vi "BoilerTimer.vi"(8 "error in (no error)":errorcluster, 10 "Enum":T1, 11 "Timer in":dbl) -> (0 "error out":errorcluster, 2 "Timer Up":bool, 3 "Elapsed Time":dbl)   [LabVIEW 2020]
uses:
  BoilerTimerStates.ctl
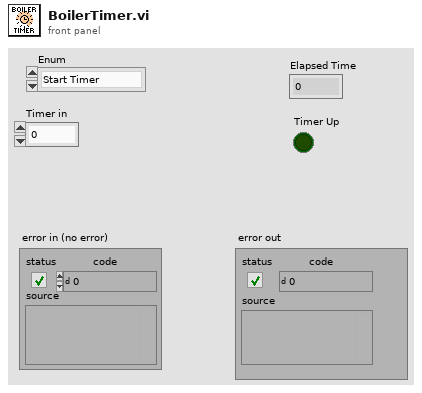
[diagram p1: front panel]
types:
  T1 = typedef "BoilerTimerStates.ctl" = enum16{"Start Timer", "Check Timer"}
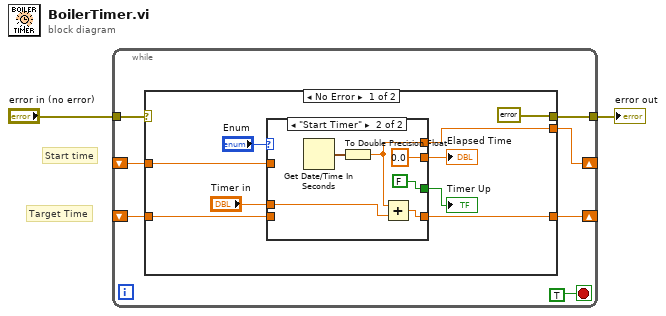
[diagram p0: block diagram]
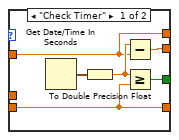
[diagram p2: hidden frame]
diagram:
  # "Target Time"
  # "Start time"
  n1 = while {
    shift-right: [w8] -> _
    shift-left: _ -> [w9]
    shift-right: [w7] -> _
    shift-left: _ -> [w6]
    tunnel: "error in (no error)" -> [w4]
    tunnel: [w3] -> w1
    stop <- TRUE stop-if-true
    n2 = case shown="No Error" w4 {
      selector: w4 -> [_ w33]
      tunnel: w9 -> [w18 w31]
      tunnel: [w17 w31] -> w8
      tunnel: [w12 w32] -> w7
      tunnel: w6 -> [w11 w32]
      tunnel: [errorcluster {"status"=FALSE, "code"=0, "source"=""} ("error IO") w33] -> w3
      frame No Error {
        n3 = case shown="\"Start Timer\"" "Enum" {
          tunnel: "Timer in" -> [_ w26]
          tunnel: [w20 w27] -> w17
          tunnel: w18 -> [w20 _]
          tunnel: [w21 0.0] -> w16
          tunnel: [w24 FALSE] -> w15
          tunnel: [w19 w25] -> w12
          tunnel: w11 -> [w19 _]
          frame "Check Timer" {
            n4 = Get Date/Time In Seconds() -> (seconds since 1Jan1904=w23:timestamp)
            n5 = To Double Precision Float(number=w23) -> (double precision float=w22:dbl)
            n6 = Subtract(x=w22, y=w20) -> (x-y=w21:dbl)
            n7 = Greater Or Equal?(x=w22, y=w19) -> (x >= y?=w24:bool)
          }
          frame "Start Timer" {
            n8 = Get Date/Time In Seconds() -> (seconds since 1Jan1904=w30:timestamp)
            n9 = To Double Precision Float(number=w30) -> (double precision float=w27:dbl)
            n10 = Add(x=w27, y=w26) -> (x+y=w25:dbl)
          }
        }
        "Timer Up" <- w15
        "Elapsed Time" <- w16
      }
      frame Error {
      }
    }
  }
  "error out" <- w1
